vi "HMS_Firmware_Manager_II.vi"(5 "error in (no error)":errorcluster) -> (13 "Pass":bool, 14 "standard error":string, 15 "standard output":string, 16 "Network Changed":bool, 17 "Module Detected":bool, 18 "Latest Firmware Found":bool, 19 "error out":errorcluster)   [LabVIEW 2025]
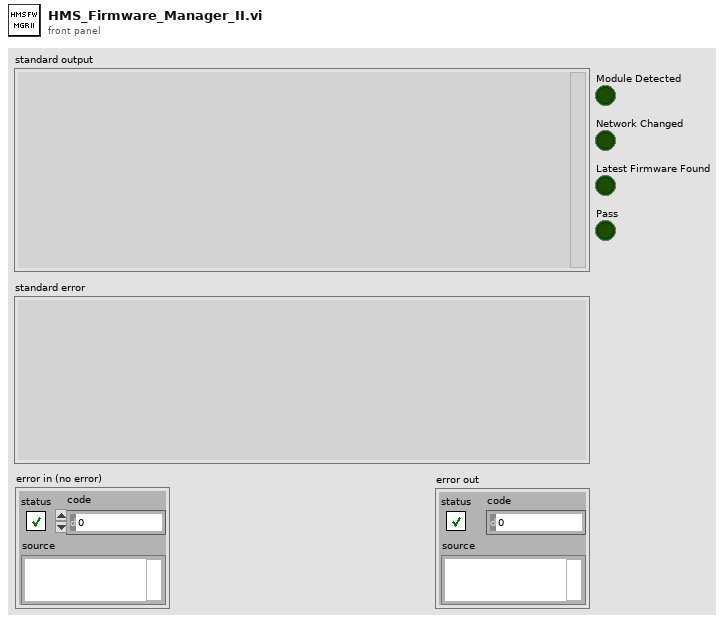
[diagram p1: front panel]
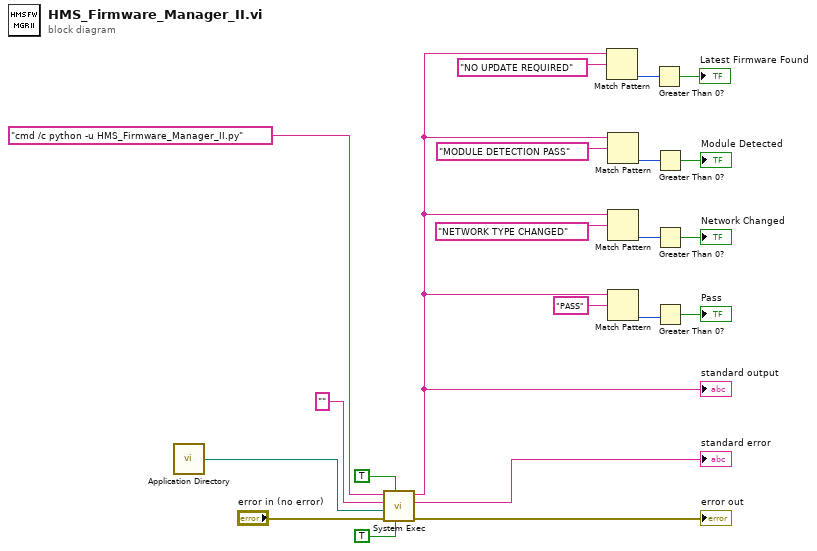
[diagram p0: block diagram]
diagram:
  n1 = call <vilib>:"Application Directory.vi"() -> ("Application Directory"=w1:path)
  n2 = call <vilib>:"System Exec.vi"("run minimized? (F)"=TRUE, "wait until completion? (T)"=TRUE ("run minimized? (F)"), "error in (no error)"="error in (no error)", "working directory"=w1, "standard input"="", "command line"="cmd /c python -u HMS_Firmware_Manager_II.py" ("name or relative path")) -> ("error out"=→"error out":errorcluster, "standard error"=→"standard error":string, "standard output"=w2:string)  [unwired: 2 in, 1 out]
  "standard output" <- w2
  n3 = Match Pattern(string=w2, regular expression="NO UPDATE REQUIRED") -> (offset past match=w5:i32)  [unwired: 1 in, 3 out]
  n4 = Match Pattern(string=w2, regular expression="MODULE DETECTION PASS") -> (offset past match=w8:i32)  [unwired: 1 in, 3 out]
  n5 = Match Pattern(string=w2, regular expression="NETWORK TYPE CHANGED") -> (offset past match=w9:i32)  [unwired: 1 in, 3 out]
  n6 = Match Pattern(string=w2, regular expression="PASS") -> (offset past match=w14:i32)  [unwired: 1 in, 3 out]
  n7 = Greater Than 0?(x=w5) -> (x > 0?=→"Latest Firmware Found":bool)
  n8 = Greater Than 0?(x=w8) -> (x > 0?=→"Module Detected":bool)
  n9 = Greater Than 0?(x=w9) -> (x > 0?=→"Network Changed":bool)
  n10 = Greater Than 0?(x=w14) -> (x > 0?=→"Pass":bool)
